vi "(SubVI) Calculate time.vi"(3 "dt":dbl, 4 "BM":dbl[](array[numeric])) -> (1 "Time (s)":dbl[](array[numeric]))   [LabVIEW 2016]
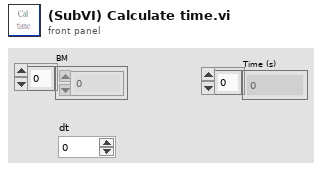
[diagram p1: front panel]
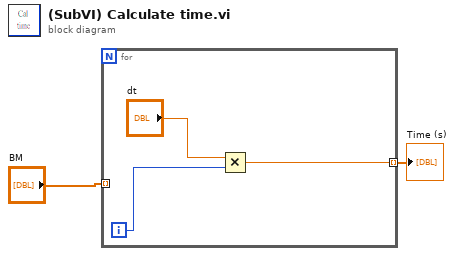
[diagram p0: block diagram]
diagram:
  n1 = for {
    tunnel: "BM" -> [_] mode=indexing
    tunnel: [w3] -> w1 mode=indexing
    i -> [w5]
    n2 = Multiply(x="dt", y=w5) -> (x*y=w3:dbl)
  }
  "Time (s)" <- w1
